vi "Untitled 3 (SubVI).vi"   [LabVIEW 2015]
types:
  T1 = typedef "WPI_EncoderDevRef.ctl" = cluster{"DevStatus":errorcluster, "EncoderIndex":T2, "CounterIndex":T3, "DistancePerCount":dbl, "Decoding Type":T4}
  T2 = typedef "FPGA_EncoderIdx.ctl" = enum8{"Enc 0", "Enc 1", "Enc 2", "Enc 3", "Enc 4", "Enc 5", "Enc 6", "Enc 7", "Invalid"}
  T3 = typedef "FPGA_CounterCtrSystemIndex.ctl" = enum8{"Ctr 0", "Ctr 1", "Ctr 2", "Ctr 3", "Ctr 4", "Ctr 5", "Ctr 6", "Ctr 7", "Invalid"}
  T4 = typedef "WPI_EncoderType.ctl" = enum16{"1x", "2x", "4x"}
  T5 = typedef "WPI_MotorControlDeviceRef.ctl" = cluster{"DeviceStatus":errorcluster, "Type":T6, "PWM":cluster{"PWM Channel":T7, "DeadBand":T8}, "CAN":cluster{"Device Number":u8, "Control Mode":T9, "Semaphore":T10, "Max Vout":dbl, "TalonSRX Control Mode":T11}, "Invert":bool}
  T6 = typedef "WPI_MotorControlType.ctl" = enum16{"PWM", "CAN", "CANTalonSRX"}
  T7 = typedef "FPGA_DIOPWMChannel.ctl" = enum8{"PWM 0", "PWM 1", "PWM 2", "PWM 3", "PWM 4", "PWM 5", "PWM 6", "PWM 7", "PWM 8", "PWM 9", "PWM MXP 0", "PWM MXP 1", "PWM MXP 2", "PWM MXP 3", "PWM MXP 4", "PWM MXP 5", "PWM MXP 6", "PWM MXP 7", "PWM MXP 8", "PWM MXP 9", "Invalid"}
  T8 = typedef "WPI_PWMDeadband.ctl" = cluster{"Name":string, "maxPositivePwm":i32, "minPositivePwm":i32, "centerPwm":i32, "maxNegativePwm":i32, "minNegativePwm":i32, "angularRange":u16}
  T9 = typedef "WPI_CANJaguar_ControlMode.ctl" = enum8{"Percent VBus", "Current", "Speed", "Position", "Voltage"}
  T10 = typedef "Semaphore RefNum" = refnum<k1>
  T11 = typedef "WPI_CANTalonSRX_APIControlMode.ctl" = enum8{"Percent VBus", "Speed", "Position", "Slave", "Unchanged / Invalid", "Voltage Compensation", "Current", "Motion Profile"}
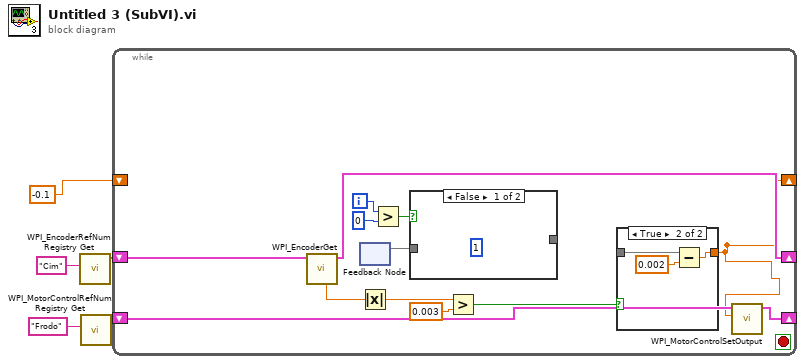
[diagram p0: block diagram]
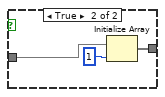
[diagram p2: hidden frame]
diagram:
  n1 = call <vilib>:"WPI_EncoderRefNum Registry Get.vi"("refnum name"="Cim") -> ("EncoderDevRef"=w4:T1)  [unwired: 9 in, 1 out]
  n2 = call <vilib>:"WPI_MotorControlRefNum Registry Get.vi"("refnum name"="Frodo") -> ("MotorControlDevRef"=w5:T5)  [unwired: 9 in, 1 out]
  n3 = while {
    shift-right: [w9] -> _
    shift-left: w4 -> [w20]
    shift-right: [w10] -> _
    shift-left: w5 -> [w15]
    shift-right: [w6] -> _
    shift-left: -0.1 -> [w7]
    i -> [w14]
    stop <- _ stop-if-true
    n4 = call <vilib>:"WPI_EncoderGet.vi"("EncoderDevRef"=w20) -> ("EncoderDevRef"=w9:T1, "Rate"=w18:dbl)  [unwired: 5 in, 4 out]
    n5 = feedback-in #1() -> (w8)
    n6 = feedback #1() -> (w11)  [unwired: 1 in]
    n7 = Absolute Value(x=w18) -> (abs(x)=w17:dbl)
    n8 = Greater?(x=w14, y=0) -> (0:w12:bool)
    n9 = case shown="False" w12 {
      tunnel: [_ w21] -> _
      tunnel: w11 -> [_ w23]
      frame False {
        (unwired) 1
      }
      frame True {
        n10 = Initialize Array(w23, 1 ("dimension size")) -> (w21:void[])
      }
    }
    n11 = Greater?(x=w17, y=0.003) -> (0:w16:bool)
    n12 = case shown="True" w16 {
      tunnel: _ -> [w24 w27]
      tunnel: [w24 w25] -> w6
      frame False {
      }
      frame True {
        n13 = Subtract(x=w27, y=0.002) -> (x-y=w25:dbl)
      }
    }
    n14 = call <vilib>:"WPI_MotorControlSetOutput.vi"("Output"=w6, "MotorControlDevRef"=w15) -> ("MotorControlDevRef"=w10:T5)  [unwired: 7 in, 2 out]
  }
